vi "Write Address Bit.vi"(8 "error in (no error)":errorcluster, 10 "Address Bit":i16[](array[numeric]), 11 "Address in":refnum<class "Address.lvclass">) -> (0 "error out":errorcluster, 3 "Address out":refnum<class "Address.lvclass">)   [LabVIEW 2020, in "Address.lvclass"]
uses:
  Address.lvclass
  Address.lvclass/Address.ctl
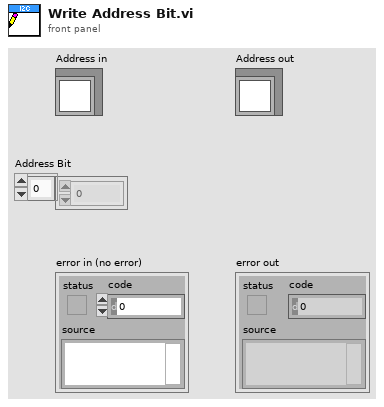
[diagram p1: front panel]
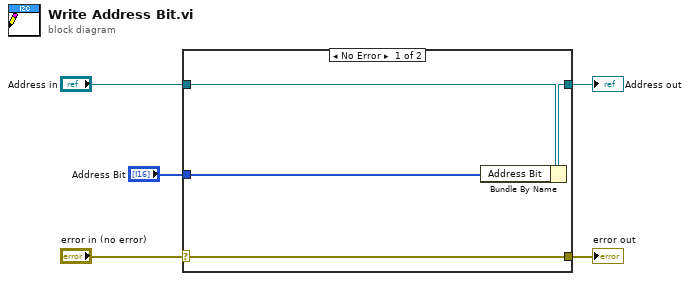
[diagram p0: block diagram]
diagram:
  n1 = case shown="No Error" "error in (no error)" {
    selector: "error in (no error)" -> [w9 w10]
    tunnel: [w9 w10] -> w4
    tunnel: [w7 w11] -> w2
    tunnel: "Address in" -> [w8 w11]
    tunnel: "Address Bit" -> [w6 _]
    frame No Error {
      n2 = Bundle By Name(cluster=w8, "Address Bit"=w6) -> (w7:refnum<class "Address.lvclass">)
    }
    frame Error {
    }
  }
  "error out" <- w4
  "Address out" <- w2
